vi "Generic - AI1.vi"(0 "MW100":refnum<visa-resource-name>="MW100", 5 "HEWH MW100 Channel Numbers":T2="A008", 11 "Error In":errorcluster, 12 "Debug":bool, 13 "Refnum in":T1) -> (4 "dup VISA session":refnum<visa-resource-name>, 6 "Value":dbl, 15 "Error Out":errorcluster)   [LabVIEW 2016]
uses:
  Type Definitions/HEWH MW100 Channel Numbers.ctl
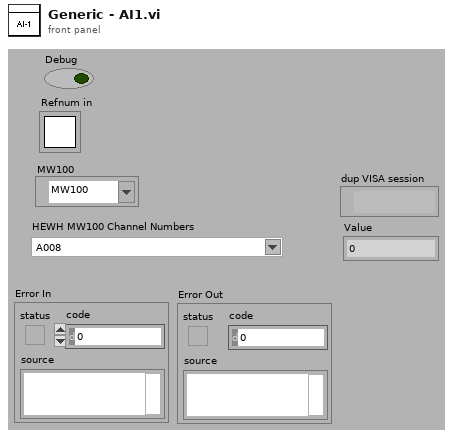
[diagram p1: front panel]
types:
  T1 = typedef "Semaphore RefNum" = refnum<k1>
  T2 = typedef "HEWH MW100 Channel Numbers.ctl" = string
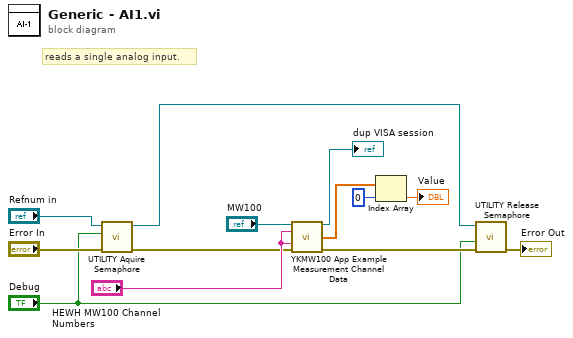
[diagram p0: block diagram]
diagram:
  # "reads a single analog input."
  n1 = call "UTILITY Aquire Semaphore.vi"("error in (no error)"="Error In", "Debug"="Debug", "Refnum in"="Refnum in") -> ("error out"=w6:errorcluster, "Refnum out"=w3:T1)  [unwired: 6 in, 1 out]
  n2 = call "YKMW100 App Example Measurement Channel Data.vi"("VISA session"="MW100", "Start Channel (001)"="HEWH MW100 Channel Numbers", "End Channel (001)"="HEWH MW100 Channel Numbers", "error in (no error)"=w6) -> ("dup VISA session"=→"dup VISA session":refnum<visa-resource-name>, "Data List"=w11:dbl[], "error out"=w5:errorcluster)  [unwired: 4 in, 5 out]
  n3 = Index Array(array=w11, index=0) -> (element=→"Value":dbl)
  n4 = call "UTILITY Release Semaphore.vi"("error in (no error)"=w5, "Debug"="Debug", "Refnum in"=w3) -> ("error out"=→"Error Out":errorcluster)  [unwired: 8 in]
